vi "RTM - Add Channels.vi"(8 "error in (no error)":errorcluster, 11 "Node Ptr":u64 format="%.0x") -> (0 "error out":errorcluster)   [LabVIEW 2019, in "UDP-Custom-Device System Explorer.lvlib"]
uses:
  UDP-Custom-Device System Explorer.lvlib
  <vilib>/NI VeriStand/Custom Device API/Custom Device Item Ref.ctl
  <vilib>/Utility/miscctls.llb/LVRowAndColumnUnsignedTypeDef.ctl
  <vilib>/NI VeriStand/Custom Device API/Custom Device Channel Type.ctl
  <vilib>/NI VeriStand/Custom Device API/Custom Device API.lvlib
  <vilib>/NI VeriStand/Custom Device Tools/Custom Device Utility Library/Custom Device Utility Library.lvlib
  Property Accessors/Shared Packet Accessors.lvlib
panel:
  in  "Remove":bool
  in  "Selected Channels":i32[](listbox)
  in  "Add":bool
  in  "Available Channels":string[](tree)
  in  "OK":bool
  in  "Cancel":bool
  in  "Initial Selection":T1[](array[typedef]) format="%.0x"
  in  "Tag":string
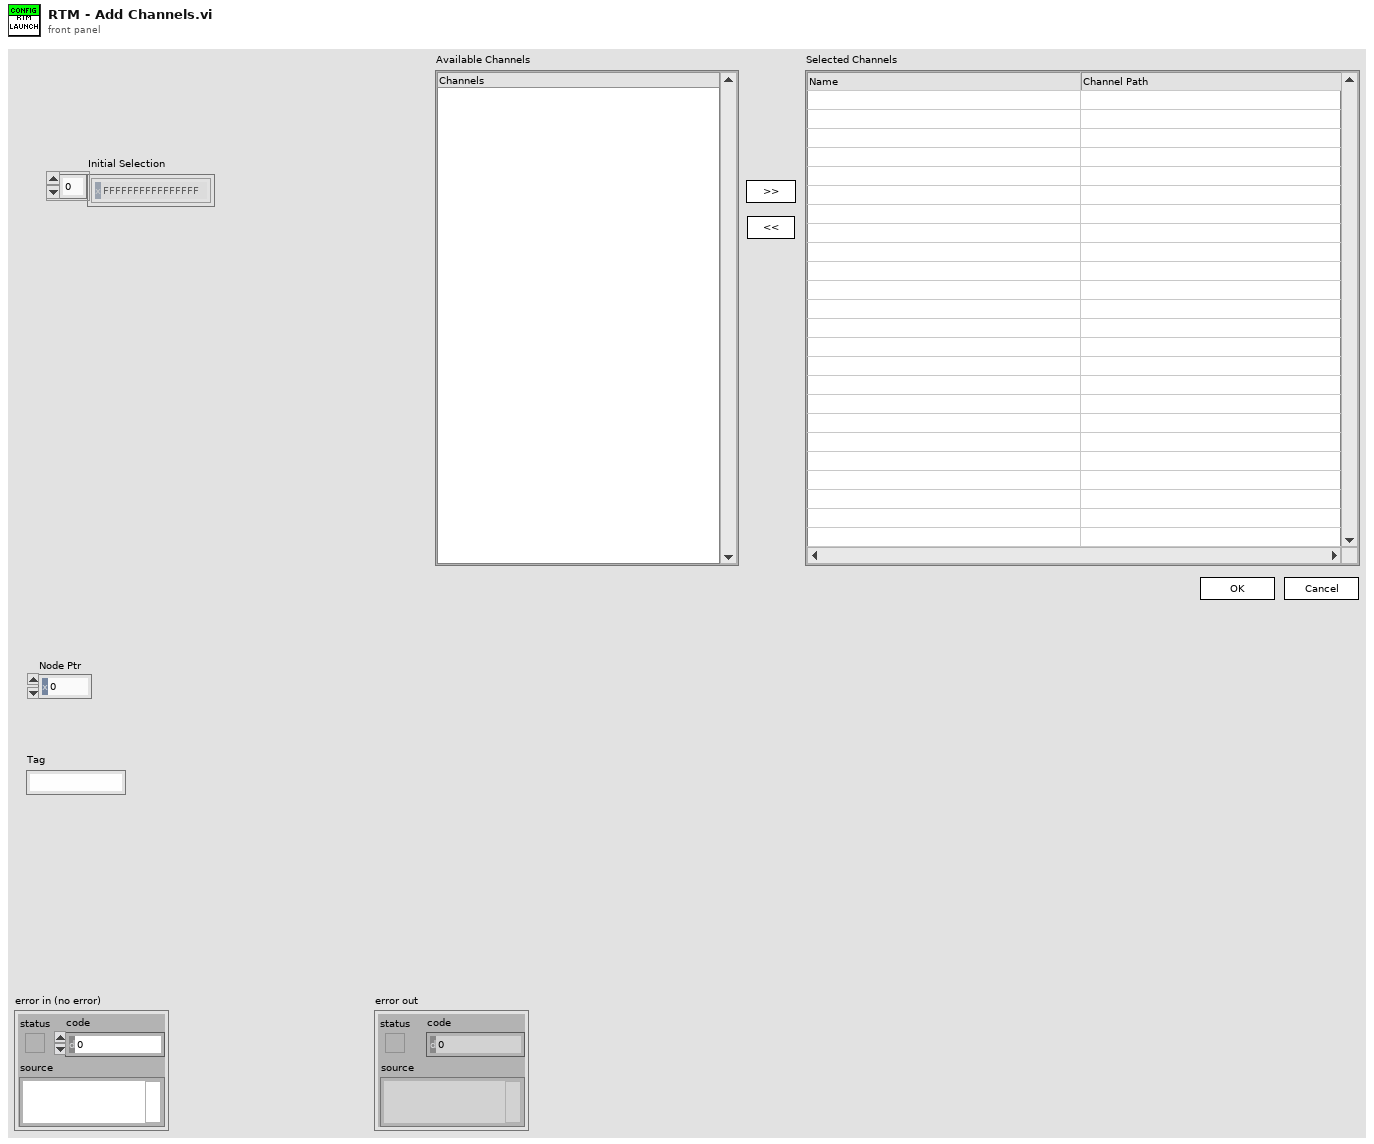
[diagram p1: front panel]
types:
  T1 = typedef "Custom Device API.lvlib/Custom Device Item Ref.ctl" = u64
  T2 = cluster{"Allow Section Selection (F)":bool, "Allow Multiple Selection (F)":bool}
  T3 = cluster{"Available Channels Label":string, "Selected Channels Label":string, "Mode":enum16{"Tx", "Rx"}}
  T4 = enum8{"Enabled", "Disabled", "Disabled and Grayed Out"}
  T5 = typedef "LVRowAndColumnUnsignedTypeDef.ctl" = cluster{"Row":u32, "Column":u32}
  T6 = typedef "Custom Device API.lvlib/Custom Device Channel Type.ctl" = enum16{"Input", "Output"}
  T7 = typedef "Custom Device API.lvlib/Custom Device Item Info.ctl" = cluster{"Name":string, "Is Channel":bool, "GUID":string, "Is Waveform":bool}
  T8 = typedef "Custom Device API.lvlib/Custom Device Channel.ctl" = cluster{"Type":T6, "Units":string, "Default Value":dbl, "Faultable":bool, "Scalable":bool}
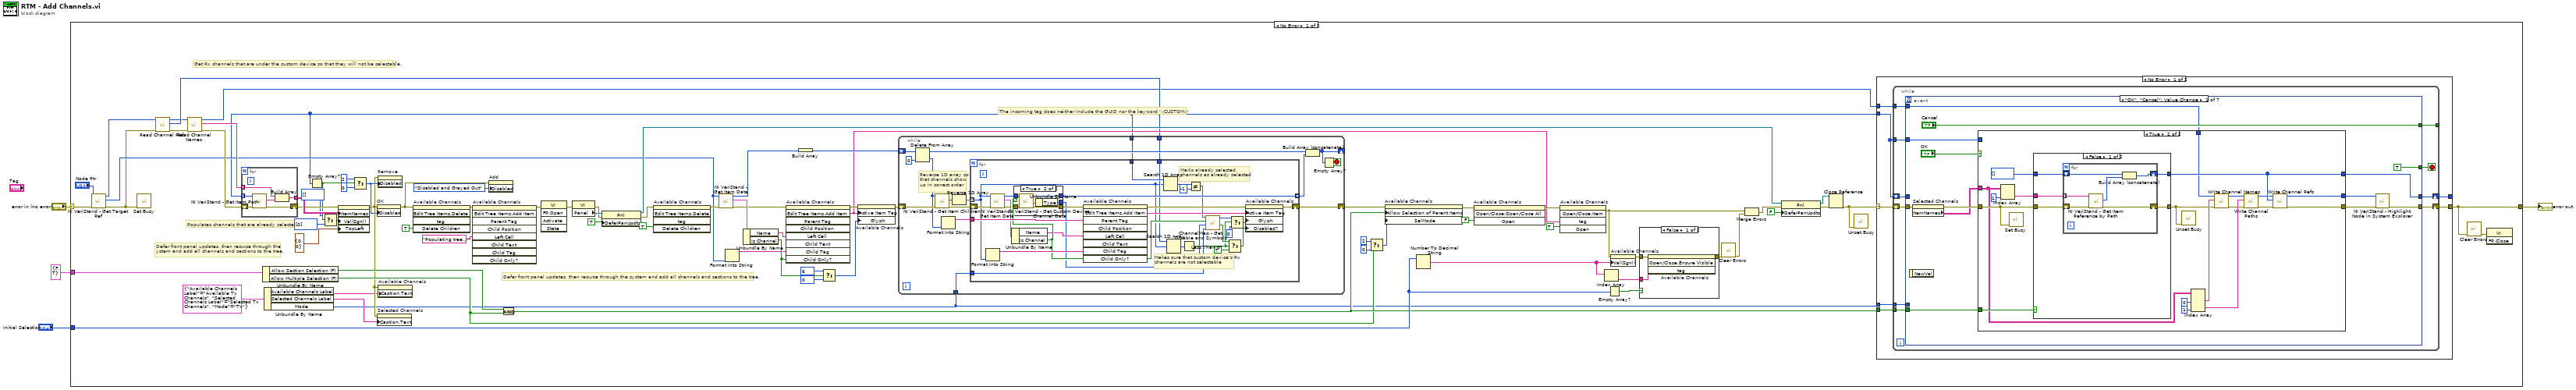
[diagram p0: block diagram]
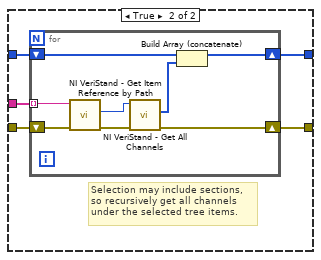
[diagram p4: hidden frame]
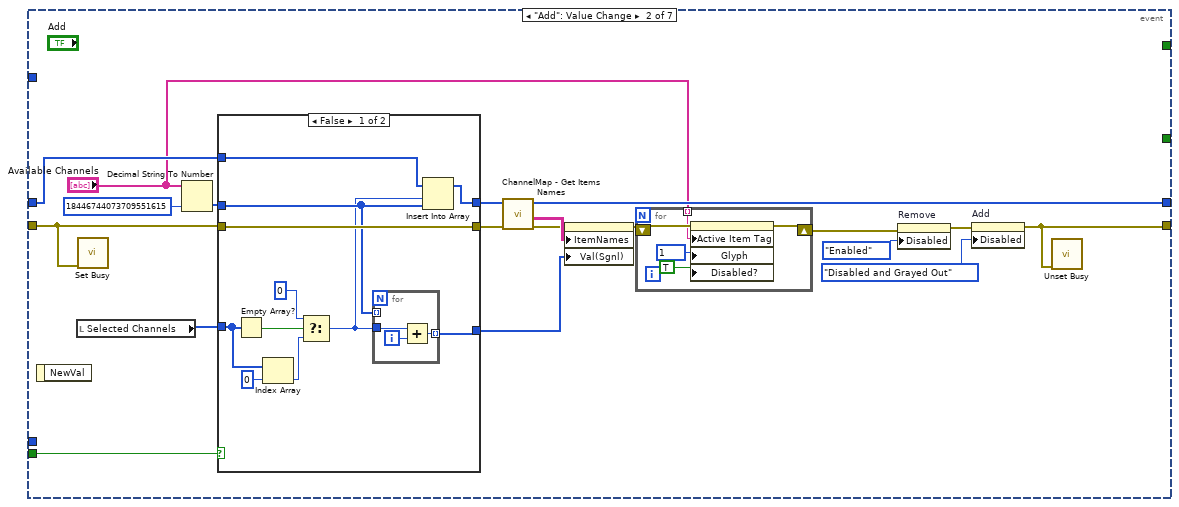
[diagram p5: hidden frame]
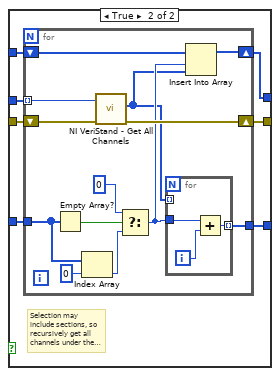
[diagram p6: hidden frame]
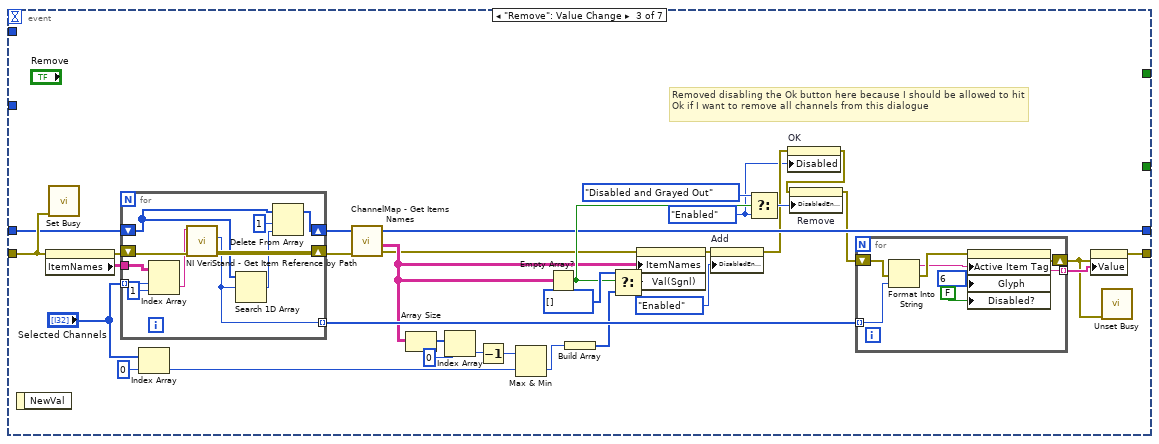
[diagram p7: hidden frame]
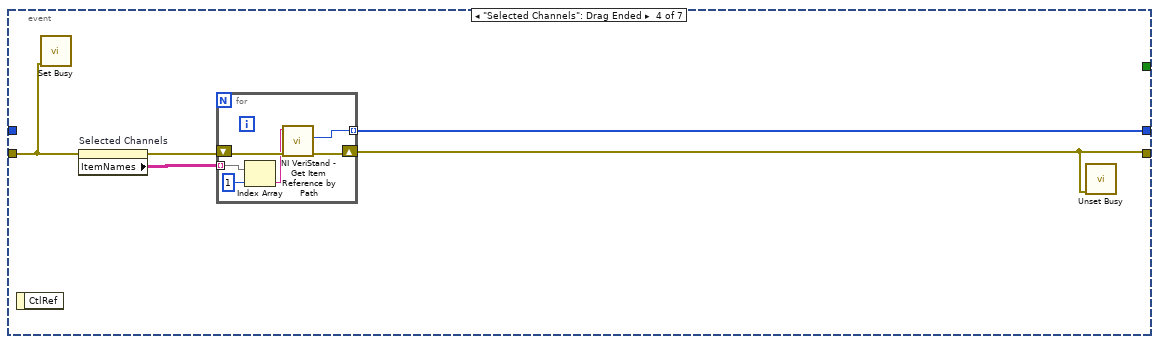
[diagram p8: hidden frame]
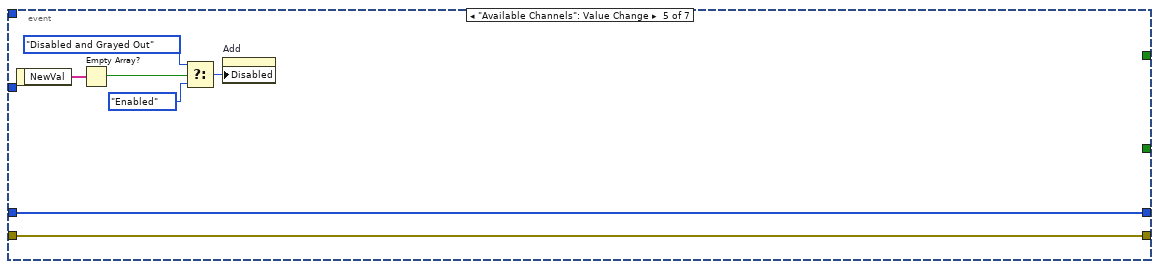
[diagram p9: hidden frame]
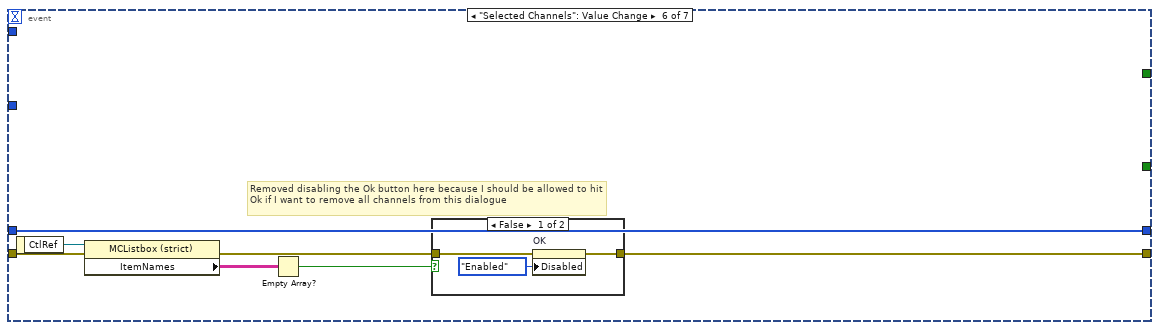
[diagram p10: hidden frame]
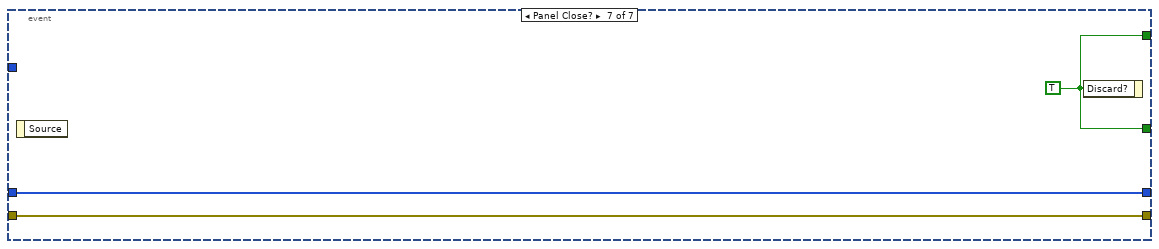
[diagram p12: hidden frame]
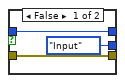
[diagram p14: hidden frame]
diagram:
  # "The incoming tag does neither include the GUID nor the keyword '::CUSTOM::'"
  n1 = case shown="No Error" "error in (no error)" {
    selector: "error in (no error)" -> [w14 w370]
    tunnel: "Initial Selection" -> [w50 _]
    tunnel: [w68 w370] -> w1
    tunnel: T2 {"Allow Section Selection (F)"=FALSE, "Allow Multiple Selection (F)"=TRUE} ("Cluster") -> [w35 _]
    frame No Error {
      # "Defer front panel updates, then recurse through the \nystem and add all channels and sections to the tree."
      # "Populates channels that are already selected"
      # "Get Rx channels that are under the custom device so that they will not be selectable."
      # "Defer front panel updates, then recurse through the system and add all channels and sections to the tree."
      n2 = call <vilib>:"NI VeriStand - Get Target Ref.vi"("error in"=w14, "Item Ref in"="Node Ptr") -> ("error out"=w10:errorcluster, "Target Ref"=w12:T1, "Item Ref out"=w11:T1)  [unwired: 6 in, 1 out]
      n3 = call <vilib>:"Set Busy.vi"("error in (no error)"=w10) -> ()  [unwired: 3 in, 8 out]
      n4 = call "Read Channel Refs.vi"("error in (no error)"=w10, "Node Ptr"=w11) -> ("error out"=w9:errorcluster, "Dependent Node Refs"=w8:T1[], "Node Ptr out"=w7:T1)  [unwired: 7 in]
      n5 = call "Read Channel Names.vi"("error in (no error)"=w9, "Node Ptr"=w7) -> ("error out"=w16:errorcluster, "Channel Names"=w15:string[], "Node Ptr out"=w6:T1)  [unwired: 7 in]
      n6 = for {
        shift-right: [w88] -> w30
        shift-left: w16 -> [w90]
        tunnel: w8 -> [w89] mode=indexing
        tunnel: [w86] -> w31 mode=indexing
        tunnel: w15 -> [w85] mode=indexing
        n7 = call <vilib>:"NI VeriStand - Get Item Path.vi"("error in (no error)"=w90, "Item Ref in"=w89) -> ("error out"=w88:errorcluster, "Path"=w87:string)  [unwired: 8 out]
        n8 = Build Array(w85, w87) -> (w86:string[])
      }
      n9 = Unbundle By Name(w35) -> ("Allow Section Selection (F)"=w34:bool, "Allow Multiple Selection (F)"=w33:bool)
      n10 = Unbundle By Name(T3 {"Available Channels Label"="Available Tx Channels", "Selected Channels Label"="Selected Tx Channels", "Mode"=enum."Tx"} ("Parameter")) -> ("Available Channels Label"=w19:string, "Selected Channels Label"=w18:string, "Mode"=w17:enum16{"Tx", "Rx"})
      n11 = Empty Array?(array=w8) -> (empty?=w24:bool)
      n12 = Select(t=i32[] [] ("Value (Signaling)"), s=w24, f=i32[] [0]) -> (s? t:f=w22:i32[])
      n13 = property on="Selected Channels" class="MCListbox (strict)"(error in=w30, "ItemNames"=w31, "Val(Sgnl)"=w22, "TopLeft"=T5 {"Row"=0, "Column"=0} ("Top Left Visible Cell")) -> (error out=w20:errorcluster)  [unwired: 1 in, 1 out]
      n14 = Select(t=u8 2, s=w24, f=u8 0) -> (s? t:f=w25:u8)
      n15 = property on="OK" class="Bool"(error in=w20, "Disabled"=w25) -> (error out=w27:errorcluster)  [unwired: 1 in, 1 out]
      n16 = property on="Selected Channels" class="MCListbox (strict)"(error in=w20, "Caption.Text"=w18) -> ()  [unwired: 1 in, 2 out]
      n17 = property on="Remove" class="Bool"(error in=w20, "Disabled"=w25) -> ()  [unwired: 1 in, 2 out]
      n18 = property on="Available Channels" class="Tree (strict)"(error in=w20, "Caption.Text"=w19) -> ()  [unwired: 1 in, 2 out]
      n19 = invoke on="Available Channels" class="Tree (strict)" method="Edit Tree Items.Delete"(error in=w27, "Delete Children"=TRUE ("Delete Children?")) -> (error out=w84:errorcluster)  [unwired: 3 in, 4 out]
      n20 = invoke on="Available Channels" class="Tree (strict)" method="Edit Tree Items.Add Item"(error in=w84, "Left Cell"="Populating tree..." ("Tag")) -> (error out=w81:errorcluster)  [unwired: 7 in, 8 out]
      n21 = property on="Add" class="Bool"(error in=w27, "Disabled"=T4."Disabled and Grayed Out") -> ()  [unwired: 1 in, 2 out]
      n22 = Compound Arithmetic op=AND(w34, w33) -> (w37:bool)
      n23 = invoke class="VI" method="FP.Open"(error in=w81) -> (error out=w79:errorcluster)  [unwired: 4 in, 4 out]
      n24 = property class="VI"(error in=w79) -> (error out=w77:errorcluster, "Panel"=w78:refnum<vi>)  [unwired: 1 in, 1 out]
      n25 = property class="Pnl"(reference=w78, error in=w77, "DeferPanUpdts"=TRUE ("Defer Panel Updates")) -> (reference out=w71:refnum<vi>, error out=w75:errorcluster)
      n26 = invoke on="Available Channels" class="Tree (strict)" method="Edit Tree Items.Delete"(error in=w75, "Delete Children"=TRUE ("Delete Children?")) -> (error out=w55:errorcluster)  [unwired: 3 in, 4 out]
      n27 = call <vilib>:"NI VeriStand - Get Item Data.vi"("error in (no error)"=w55, "Item Ref in"=w12) -> ("error out"=w58:errorcluster, "Item Info"=w60:T7, "Item Ref out"=w56:T1)  [unwired: 7 out]
      n28 = Format Into String(w12) -> (resulting string=w59:string)  [unwired: 3 in, 1 out]
      n29 = Unbundle By Name(w60) -> ("Name"=w61:string, "Is Channel"=w65:bool)
      n30 = invoke on="Available Channels" class="Tree (strict)" method="Edit Tree Items.Add Item"(error in=w58, "Left Cell"=w61, "Child Tag"=w59, "Child Only?"=w65) -> (error out=w62:errorcluster, "Edit Tree Items:Add Item"=w41:string)  [unwired: 5 in, 7 out]
      n31 = Build Array(w56) -> (w74:T1[])
      n32 = Select(t=6, s=w65, f=0) -> (s? t:f=w66:i32)
      n33 = property on="Available Channels" class="Tree (strict)"(error in=w62, "Active Item Tag"=w41, "Glyph"=w66) -> (error out=w57:errorcluster)  [unwired: 1 in, 1 out]
      n34 = while {
        shift-right: [w322] -> w73
        shift-left: w57 -> [w328]
        shift-right: [w327] -> _
        shift-left: w74 -> [w331]
        tunnel: w8 -> [w319]
        tunnel: w17 -> [w318]
        tunnel: w8 -> [w317]
        stop <- w326 stop-if-true
        # "Reverse 1D array so that channels show up in correct order"
        n35 = Delete From Array(array=w331, index=0) -> (deleted portion=w321:T1, array with subset deleted=w329:T1[])  [unwired: 1 in]
        n36 = call <vilib>:"NI VeriStand - Get Item Children.vi"("error in (no error)"=w328, "Item Ref in"=w321) -> ("error out"=w325:errorcluster, "Child Refs"=w324:T1[])  [unwired: 8 out]
        n37 = Format Into String(w321) -> (resulting string=w320:string)  [unwired: 3 in, 1 out]
        n38 = Reverse 1D Array(array=w324) -> (reversed array=w316:T1[])
        n39 = for {
          shift-right: [w354] -> w322
          shift-left: w325 -> [w359]
          tunnel: w316 -> [w341] mode=indexing
          tunnel: [w351] -> w323 mode=indexing
          tunnel: w320 -> [w360]
          tunnel: w319 -> [w353]
          tunnel: w318 -> [w345]
          tunnel: w317 -> [w342]
          # "Marks already selected channels as already selected"
          # "Makes sure that custom device's Rx channels are not selectable"
          n40 = Format Into String(w341) -> (resulting string=w358:string)  [unwired: 3 in, 1 out]
          n41 = call <vilib>:"NI VeriStand - Get Item Data.vi"("error in (no error)"=w359, "Item Ref in"=w341) -> ("error out"=w350:errorcluster, "Item Info"=w357:T7, "Item Ref out"=w352:T1)  [unwired: 7 out]
          n42 = Unbundle By Name(w357) -> ("Name"=w343:string, "Is Channel"=w344:bool)
          n43 = case shown="True" w344 {
            tunnel: w352 -> [w363 w369]
            tunnel: [w363 w368] -> w351
            tunnel: w350 -> [w362 w367]
            tunnel: [w362 w366] -> w349
            tunnel: [Custom_Device_Channel_Type."Input" ("Type") w364] -> w339
            frame False {
            }
            frame True {
              n44 = call <vilib>:"NI VeriStand - Get Custom Device Channel Data.vi"("error in (no error)"=w367, "Channel Ref in"=w369) -> ("error out"=w366:errorcluster, "Channel"=w365:T8, "Channel Ref out"=w368:T1)  [unwired: 4 in, 3 out]
              n45 = Unbundle By Name(w365) -> ("Type"=w364:T6)
            }
          }
          n46 = invoke on="Available Channels" class="Tree (strict)" method="Edit Tree Items.Add Item"(error in=w349, "Parent Tag"=w360, "Left Cell"=w343, "Child Tag"=w358, "Child Only?"=w344) -> (error out=w356:errorcluster, "Edit Tree Items:Add Item"=w355:string)  [unwired: 4 in, 7 out]
          n47 = Search 1D Array(1D array=w353, element=w341) -> (index of element=w348:i32)  [unwired: 1 in]
          n48 = Search 1D Array(1D array=w342, element=w341) -> (index of element=w340:i32)  [unwired: 1 in]
          n49 = Less Than 0?(x=w340) -> (x < 0?=w333:bool)
          n50 = Not Equal?(x=w348, y=-1) -> (x != y?=w346:bool)
          n51 = call "ChannelMap - Get Disable and Symbols.vi"("Mode"=w345, "Channel Type"=w339, "Is Channel?"=w344, "Is Selected?"=w346) -> ("Disabled?"=w338:bool, "Symbole"=w335:i32)  [unwired: 6 in]
          n52 = Select(t=w338, s=w333, f=TRUE) -> (s? t:f=w337:bool)
          n53 = Select(t=w335, s=w333, f=0) -> (s? t:f=w334:i32)
          n54 = property on="Available Channels" class="Tree (strict)"(error in=w356, "Active Item Tag"=w355, "Glyph"=w334, "Disabled?"=w337) -> (error out=w354:errorcluster)  [unwired: 1 in, 1 out]
        }
        n55 = Build Array (concatenate)(w329, w323) -> (w327:T1[])
        n56 = Empty Array?(array=w327) -> (empty?=w326:bool)
      }
      n57 = Select(t=2 ("Selection Mode"), s=w33, f=0 ("Selection Mode")) -> (s? t:f=w38:i32)
      n58 = property on="Available Channels" class="Tree (strict)"(error in=w73, "Allow Selection of Parent Items"=w37, "SelMode"=w38) -> (error out=w46:errorcluster)  [unwired: 1 in, 1 out]
      n59 = Number To Decimal String(number=w50) -> (decimal integer string=w48:string[])  [unwired: 1 out]
      n60 = invoke on="Available Channels" class="Tree (strict)" method="Open/Close.Open/Close All"(error in=w46, "Open"=FALSE ("Open?")) -> (error out=w44:errorcluster)  [unwired: 2 in, 3 out]
      n61 = invoke on="Available Channels" class="Tree (strict)" method="Open/Close.Item"(error in=w44, "tag"=w41, "Open"=TRUE ("Open?")) -> (error out=w42:errorcluster)  [unwired: 2 in, 4 out]
      n62 = Index Array(array=w48) -> (element=w47:string)  [unwired: 1 in]
      n63 = Empty Array?(array=w50) -> (empty?=w49:bool)
      n64 = property on="Available Channels" class="Tree (strict)"(error in=w42, "Val(Sgnl)"=w48) -> (error out=w52:errorcluster)  [unwired: 1 in, 1 out]
      n65 = case shown="False" w49 {
        tunnel: w52 -> [w93 w94]
        tunnel: [w92 w94] -> w51
        tunnel: w47 -> [w91 _]
        frame False {
          n66 = invoke on="Available Channels" class="Tree (strict)" method="Open/Close.Ensure Visible"(error in=w93, "tag"=w91) -> (error out=w92:errorcluster)  [unwired: 2 in, 3 out]
        }
        frame True {
        }
      }
      n67 = call <vilib>:"Clear Errors.vi"("error in (no error)"=w51) -> ("error out"=w54:errorcluster)  [unwired: 1 in, 5 out]
      n68 = Merge Errors(w42, w54) -> (w53:errorcluster)
      n69 = property class="Pnl"(reference=w71, error in=w53, "DeferPanUpdts"=FALSE ("Defer Panel Updates")) -> (reference out=w69:refnum<vi>, error out=w70:errorcluster)
      n70 = Close Reference(reference=w69, error in (no error)=w70) -> (error out=w36:errorcluster)
      n71 = call <vilib>:"Unset Busy.vi"("error in (no error)"=w36) -> ()  [unwired: 1 in, 10 out]
      n72 = case shown="No Error" w36 {
        selector: w36 -> [w101 w315]
        tunnel: [w100 w315] -> w68
        tunnel: [w99 w314] -> _
        tunnel: w37 -> [w98 _]
        tunnel: w8 -> [w97 w314]
        tunnel: w17 -> [w96 _]
        tunnel: w6 -> [w95 _]
        frame No Error {
          n73 = while {
            shift-right: [w110] -> w100
            shift-left: w101 -> [w111]
            tunnel: [w109] -> _
            tunnel: w98 -> [w107]
            shift-right: [w104] -> w99
            shift-left: w97 -> [w106]
            tunnel: w97 -> [w105]
            tunnel: w96 -> [w103]
            tunnel: w95 -> [w102]
            stop <- w108 stop-if-true
            n74 = event shown="[0] \"OK\", \"Cancel\": Value Change" {
              selector: _ -> [_ _ _ _ _ _ _]
              dyn-events: _ -> [_ _ _ _ _ _ _]
              timeout: _ -> [_ _ _ _ _ _ _]
              tunnel: w111 -> [w120 w187 w263 w286 w299 w304 w313]
              tunnel: [w116 w171 w236 w283 w299 w301 w313] -> w110
              tunnel: ["Cancel" _ _ _ _ _ w312] -> w109
              tunnel: [TRUE ("Discard?") _ _ _ _ _ w312] -> w108
              tunnel: [w112 w183 w242 w282 w296 w306 w311] -> w104
              tunnel: w107 -> [w122 w186 _ _ _ _ _]
              tunnel: w106 -> [_ w185 w260 _ w296 w306 w311]
              tunnel: w105 -> [w118 _ _ _ _ _ _]
              tunnel: w103 -> [_ _ _ _ _ _ _]
              tunnel: w102 -> [w115 _ _ _ _ _ _]
              event "OK", "Cancel": Value Change {
                n75 = event-data() -> ()  [unwired: 2 out]
                n76 = property on="Selected Channels" class="MCListbox (strict)"(error in=w120) -> (error out=w119:errorcluster, "ItemNames"=w117:string[][])  [unwired: 1 in, 1 out]
                n77 = case shown="True" "OK" {
                  tunnel: w117 -> [_ w139]
                  tunnel: w122 -> [_ w146]
                  tunnel: w119 -> [w127 w144]
                  tunnel: [w126 w138] -> w112
                  tunnel: [w127 w137] -> w113
                  tunnel: w118 -> [w126 _]
                  tunnel: w115 -> [w125 w135]
                  tunnel: [w125 w136] -> w114
                  frame False {
                  }
                  frame True {
                    n78 = Index Array(array=w139, index (col)=1 ("disabled index (col)")) -> (element=w142:string[])  [unwired: 1 in]
                    n79 = call <vilib>:"Set Busy.vi"("error in (no error)"=w144) -> ()  [unwired: 3 in, 8 out]
                    n80 = case shown="False" w146 {
                      tunnel: w144 -> [w151 w162]
                      tunnel: [w147 w160] -> w138
                      tunnel: [w150 w159] -> w133
                      tunnel: T1[] [] ("Channel Refs") -> [w148 w161]
                      tunnel: w142 -> [w149 w158]
                      frame False {
                        n81 = for {
                          tunnel: w149 -> [w155] mode=indexing
                          shift-right: [w152] -> w147
                          shift-left: w148 -> [w153]
                          shift-right: [w156] -> w150
                          shift-left: w151 -> [w157]
                          n82 = call <vilib>:"NI VeriStand - Get Item Reference by Path.vi"("error in (no error)"=w157, "Item Path in"=w155) -> ("error out"=w156:errorcluster, "Item Ref"=w154:T1)  [unwired: 6 in, 2 out]
                          n83 = Build Array (concatenate)(w153, w154) -> (w152:T1[])
                        }
                      }
                      frame True {
                        # "Selection may include sections, so recursively get all channels under the selected tree items."
                        n84 = for {
                          shift-right: [w168] -> w160
                          shift-left: w161 -> [w169]
                          shift-right: [w170] -> w159
                          shift-left: w162 -> [w165]
                          tunnel: w158 -> [w166] mode=indexing
                          n85 = call <vilib>:"NI VeriStand - Get Item Reference by Path.vi"("error in (no error)"=w165, "Item Path in"=w166) -> ("error out"=w164:errorcluster, "Item Ref"=w163:T1)  [unwired: 6 in, 2 out]
                          n86 = call <vilib>:"NI VeriStand - Get All Channels.vi"("error in"=w164, "Section Ref in"=w163) -> ("error out"=w170:errorcluster, "Channel Refs"=w167:T1[])  [unwired: 8 out]
                          n87 = Build Array (concatenate)(w169, w167) -> (w168:T1[])
                        }
                      }
                    }
                    n88 = call <vilib>:"Unset Busy.vi"("error in (no error)"=w133) -> ()  [unwired: 1 in, 10 out]
                    n89 = Index Array(array=w139, index (col) #1=0 ("disabled index (col)"), index (col) #2=1 ("index (col)")) -> (element #1=w134:string[], element #2=w131:string[])  [unwired: 2 in]
                    n90 = call "Write Channel Names.vi"("error in (no error)"=w133, "Channel Names"=w134, "Node Ptr"=w135) -> ("error out"=w130:errorcluster, "Node Ptr out"=w132:T1)  [unwired: 7 in]
                    n91 = call "Write Channel Paths.vi"("error in (no error)"=w130, "Channel Paths"=w131, "Node Ptr"=w132) -> ("error out"=w129:errorcluster, "Node Ptr out"=w128:T1)  [unwired: 7 in]
                    n92 = call "Write Channel Refs.vi"("error in (no error)"=w129, "Dependent Node Refs"=w138, "Node Ptr"=w128) -> ("error out"=w137:errorcluster, "Node Ptr out"=w136:T1)  [unwired: 7 in]
                  }
                }
                n93 = call <vilib>:"NI VeriStand - Highlight Node in System Explorer.vi"("error in (no error)"=w113, "Item Ref in"=w114) -> ("error out"=w116:errorcluster)  [unwired: 8 in, 1 out]
              }
              event "Add": Value Change {
                n94 = event-data() -> ()  [unwired: 2 out]
                n95 = local read "Selected Channels"() -> (w175:i32[])
                n96 = call <vilib>:"Set Busy.vi"("error in (no error)"=w187) -> ()  [unwired: 3 in, 8 out]
                n97 = Decimal String To Number(string="Available Channels", default (0L)=T1 18446744073709551615 ("Device Item Ref")) -> (number=w189:u64[])  [unwired: 2 out]
                n98 = case shown="False" w186 {
                  tunnel: w187 -> [w205 w215]
                  tunnel: [w202 w214] -> w184
                  tunnel: w189 -> [w197 w213]
                  tunnel: [w205 w212] -> w182
                  tunnel: w185 -> [w203 w211]
                  tunnel: w175 -> [w201 w210]
                  tunnel: [w195 w209] -> w174
                  frame False {
                    n99 = Empty Array?(array=w201) -> (empty?=w204:bool)
                    n100 = Index Array(array=w201, index=0) -> (element=w199:i32)
                    n101 = Select(t=0, s=w204, f=w199) -> (s? t:f=w196:i32)
                    n102 = for {
                      tunnel: w197 -> [_] mode=indexing
                      tunnel: w196 -> [w208]
                      tunnel: [w206] -> w195 mode=indexing
                      i -> [w207]
                      n103 = Add(x=w208, y=w207) -> (x+y=w206:i32)
                    }
                    n104 = Insert Into Array(array=w203, index=w196, new element=w197) -> (w202:T1[])
                  }
                  frame True {
                    # "Selection may include sections, so recursively get all channels under the selected tree items."
                    n105 = for {
                      shift-right: [w220] -> w214
                      shift-left: w211 -> [w219]
                      shift-right: [w227] -> w212
                      shift-left: w215 -> [w228]
                      tunnel: w213 -> [w226] mode=indexing
                      tunnel: w210 -> [w221]
                      tunnel: [w218] -> w209
                      n106 = Empty Array?(array=w221) -> (empty?=w222:bool)
                      n107 = Index Array(array=w221, index=0) -> (element=w224:i32)
                      n108 = call <vilib>:"NI VeriStand - Get All Channels.vi"("error in"=w228, "Section Ref in"=w226) -> ("error out"=w227:errorcluster, "Channel Refs"=w216:T1[])  [unwired: 8 out]
                      n109 = Select(t=0, s=w222, f=w224) -> (s? t:f=w217:i32)
                      n110 = for {
                        tunnel: w217 -> [w231]
                        tunnel: [w229] -> w218 mode=indexing
                        tunnel: w216 -> [_] mode=indexing
                        i -> [w230]
                        n111 = Add(x=w231, y=w230) -> (x+y=w229:i32)
                      }
                      n112 = Insert Into Array(array=w219, index=w217, new element=w216) -> (w220:T1[])
                    }
                  }
                }
                n113 = call "ChannelMap - Get Items Names.vi"("error IO 2"=w182, "TCP Channel Refs In"=w184) -> ("error IO"=w177:errorcluster, "Items Names"=w178:string[][], "TCP Channel Refs Out"=w183:T1[])  [unwired: 7 in]
                n114 = property on="Selected Channels" class="MCListbox (strict)"(error in=w177, "ItemNames"=w178, "Val(Sgnl)"=w174) -> (error out=w181:errorcluster)  [unwired: 1 in, 1 out]
                n115 = for {
                  shift-right: [w193] -> w173
                  shift-left: w181 -> [w194]
                  tunnel: "Available Channels" -> [w191] mode=indexing
                  n116 = property on="Available Channels" class="Tree (strict)"(error in=w194, "Active Item Tag"=w191, "Glyph"=1, "Disabled?"=TRUE ("Active Item:Disabled?")) -> (error out=w193:errorcluster)  [unwired: 1 in, 1 out]
                }
                n117 = property on="Remove" class="Bool"(error in=w173, "Disabled"=T4."Enabled") -> (error out=w172:errorcluster)  [unwired: 1 in, 1 out]
                n118 = property on="Add" class="Bool"(error in=w172, "Disabled"=T4."Disabled and Grayed Out") -> (error out=w171:errorcluster)  [unwired: 1 in, 1 out]
                n119 = call <vilib>:"Unset Busy.vi"("error in (no error)"=w171) -> ()  [unwired: 1 in, 10 out]
              }
              event "Remove": Value Change {
                w233 = T4."Enabled" ("Disabled")
                # "Removed disabling the Ok button here because I should be allowed to hit Ok if I want to remove all channels from this dialogue"
                n120 = event-data() -> ()  [unwired: 2 out]
                n121 = property on="Selected Channels" class="MCListbox (strict)"(error in=w263) -> (error out=w262:errorcluster, "ItemNames"=w261:string[][])  [unwired: 1 in, 1 out]
                n122 = call <vilib>:"Set Busy.vi"("error in (no error)"=w263) -> ()  [unwired: 3 in, 8 out]
                n123 = for {
                  tunnel: w261 -> [w272]
                  tunnel: "Selected Channels" -> [w273] mode=indexing
                  shift-right: [w271] -> w244
                  shift-left: w262 -> [w274]
                  shift-right: [w269] -> w241
                  shift-left: w260 -> [w270]
                  tunnel: [w266] -> w259 mode=indexing
                  n124 = Index Array(array=w272, index (row)=w273, index (col)=1 ("disabled index (col)")) -> (element=w264:string)
                  n125 = call <vilib>:"NI VeriStand - Get Item Reference by Path.vi"("error in (no error)"=w274, "Item Path in"=w264) -> ("error out"=w271:errorcluster, "Item Ref"=w266:T1)  [unwired: 6 in, 2 out]
                  n126 = Search 1D Array(1D array=w270, element=w266) -> (index of element=w267:i32)  [unwired: 1 in]
                  n127 = Delete From Array(array=w270, length=1, index=w267) -> (array with subset deleted=w269:T1[])  [unwired: 1 out]
                }
                n128 = Index Array(array="Selected Channels", index=0) -> (element=w247:i32)
                n129 = call "ChannelMap - Get Items Names.vi"("error IO 2"=w244, "TCP Channel Refs In"=w241) -> ("error IO"=w240:errorcluster, "Items Names"=w243:string[][], "TCP Channel Refs Out"=w242:T1[])  [unwired: 7 in]
                n130 = Array Size(array=w243) -> (size(s)=w251:i32[])
                n131 = Index Array(array=w251, index=0) -> (element=w249:i32)
                n132 = Decrement(x=w249) -> (x-1=w248:i32)
                n133 = Max & Min(x=w248, y=w247) -> (min(x,y)=w246:i32)  [unwired: 1 out]
                n134 = Empty Array?(array=w243) -> (empty?=w256:bool)
                n135 = Build Array(w246) -> (w253:i32[])
                n136 = Select(t=i32[] [] ("Selected TCP Channels"), s=w256, f=w253) -> (s? t:f=w257:i32[])
                n137 = property on="Selected Channels" class="MCListbox (strict)"(error in=w240, "ItemNames"=w243, "Val(Sgnl)"=w257) -> ()  [unwired: 1 in, 2 out]
                n138 = property on="Add" class="Bool"(error in=w240, "DisabledEnum"=T4."Enabled" ("Disabled")) -> (error out=w239:errorcluster)  [unwired: 1 in, 1 out]
                n139 = Select(t=T4."Disabled and Grayed Out" ("Disabled"), s=w256, f=w233) -> (s? t:f=w255:T4)
                n140 = property on="OK" class="Bool"(error in=w239, "Disabled"=w233) -> (error out=w238:errorcluster)  [unwired: 1 in, 1 out]
                n141 = property on="Remove" class="Bool"(error in=w238, "DisabledEnum"=w255) -> (error out=w237:errorcluster)  [unwired: 1 in, 1 out]
                n142 = for {
                  shift-right: [w279] -> w235
                  shift-left: w237 -> [w277]
                  tunnel: w259 -> [w278] mode=indexing
                  tunnel: [w275] -> w245 mode=indexing
                  n143 = Format Into String(error in=w277, w278) -> (resulting string=w275:string, error out=w276:errorcluster)  [unwired: 2 in]
                  n144 = property on="Available Channels" class="Tree (strict)"(error in=w276, "Active Item Tag"=w275, "Glyph"=6, "Disabled?"=FALSE ("Active Item:Disabled?")) -> (error out=w279:errorcluster)  [unwired: 1 in, 1 out]
                }
                n145 = property on="Available Channels" class="Tree (strict)"(error in=w235, "Value"=w245) -> (error out=w236:errorcluster)  [unwired: 1 in, 1 out]
                n146 = call <vilib>:"Unset Busy.vi"("error in (no error)"=w235) -> ()  [unwired: 1 in, 10 out]
              }
              event "Selected Channels": Drag Ended {
                n147 = event-data() -> ()  [unwired: 2 out]
                n148 = call <vilib>:"Set Busy.vi"("error in (no error)"=w286) -> ()  [unwired: 3 in, 8 out]
                n149 = property on="Selected Channels" class="MCListbox (strict)"(error in=w286) -> (error out=w285:errorcluster, "ItemNames"=w284:string[][])  [unwired: 1 in, 1 out]
                n150 = for {
                  tunnel: w284 -> [w291] mode=indexing
                  shift-right: [w290] -> w283
                  shift-left: w285 -> [w292]
                  tunnel: [w289] -> w282 mode=indexing
                  n151 = Index Array(array=w291, index=1 ("disabled index (col)")) -> (element=w288:string)
                  n152 = call <vilib>:"NI VeriStand - Get Item Reference by Path.vi"("error in (no error)"=w292, "Item Path in"=w288) -> ("error out"=w290:errorcluster, "Item Ref"=w289:T1)  [unwired: 6 in, 2 out]
                }
                n153 = call <vilib>:"Unset Busy.vi"("error in (no error)"=w283) -> ()  [unwired: 1 in, 10 out]
              }
              event "Available Channels": Value Change {
                n154 = event-data() -> ("NewVal"=w298:string[])  [unwired: 1 out]
                n155 = Empty Array?(array=w298) -> (empty?=w295:bool)
                n156 = Select(t=T4."Disabled and Grayed Out" ("Disabled"), s=w295, f=T4."Enabled" ("Disabled")) -> (s? t:f=w297:T4)
                n157 = property on="Add" class="Bool"("Disabled"=w297) -> ()  [unwired: 2 in, 2 out]
              }
              event "Selected Channels": Value Change {
                # "Removed disabling the Ok button here because I should be allowed to hit Ok if I want to remove all channels from this dialogue"
                n158 = event-data() -> ("CtlRef"=w305:refnum<vi>)  [unwired: 1 out]
                n159 = property class="MCListbox (strict)"(reference=w305, error in=w304) -> (error out=w302:errorcluster, "ItemNames"=w303:string[][])  [unwired: 1 out]
                n160 = Empty Array?(array=w303) -> (empty?=w300:bool)
                n161 = case shown="False" w300 {
                  tunnel: w302 -> [w309 w310]
                  tunnel: [w308 w310] -> w301
                  frame False {
                    n162 = property on="OK" class="Bool"(error in=w309, "Disabled"=T4."Enabled") -> (error out=w308:errorcluster)  [unwired: 1 in, 1 out]
                  }
                  frame True {
                  }
                }
              }
              event Panel Close? {
                w312 = TRUE ("Discard?")
                n163 = event-data() -> ()  [unwired: 2 out]
                n164 = event-data("Discard?"=w312) -> ()  [unwired: 1 in, 1 out]
              }
            }
          }
        }
        frame Error {
        }
      }
      n165 = call <vilib>:"Clear Errors.vi"("error in (no error)"=w68) -> ("error out"=w67:errorcluster)  [unwired: 1 in, 5 out]
      n166 = invoke class="VI" method="FP.Close"(error in=w67) -> ()  [unwired: 2 in, 3 out]
    }
    frame Error {
    }
  }
  "error out" <- w1
